vi "get piece from region 1.vi"   [LabVIEW 2018]
types:
  T1 = enum16{"shoulder", "elbow", "wrist", "base", "gripper"}
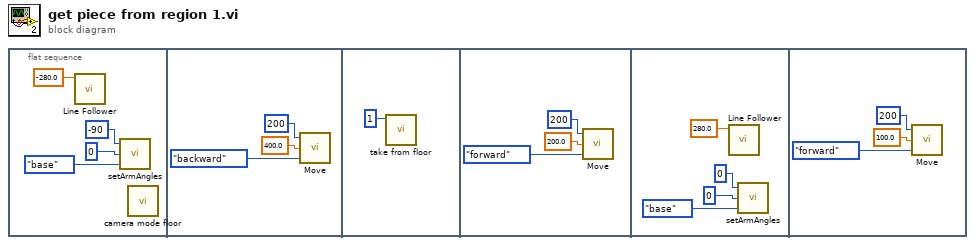
[diagram p0: block diagram]
diagram:
  n1 = flat-sequence {
    frame #0 {
      n2 = call "Line Follower.vi"("speed"=-280.0) -> ()  [unwired: 11 in]
      n3 = call "setArmAngles.vi"("Enum"=T1."base", "speed"=0, "angle"=-90) -> ()  [unwired: 1 in]
      n4 = call "camera mode floor.vi"() -> ()  [unwired: 12 in]
    }
    frame #1 {
      n5 = call "Move.vi"("Enum"=enum16{"forward", "backward", "left", "right"}."backward", "distance"=400.0, "speed"=200) -> ()  [unwired: 1 in]
    }
    frame #2 {
      n6 = call "take from floor.vi"("m"=1) -> ()  [unwired: 11 in]
    }
    frame #3 {
      n7 = call "Move.vi"("Enum"=enum16{"forward", "backward", "left", "right"}."forward", "distance"=200.0, "speed"=200) -> ()  [unwired: 1 in]
    }
    frame #4 {
      n8 = call "Line Follower.vi"("speed"=280.0) -> ()  [unwired: 11 in]
      n9 = call "setArmAngles.vi"("Enum"=T1."base", "speed"=0, "angle"=0) -> ()  [unwired: 1 in]
    }
    frame #5 {
      n10 = call "Move.vi"("Enum"=enum16{"forward", "backward", "left", "right"}."forward", "distance"=100.0, "speed"=200) -> ()  [unwired: 1 in]
    }
  }
